vi "Drive Motor TXRX.vi"(0 "Error In":errorcluster, 1 "Speed Control (m/s)":dbl, 3 "RPM / Speed":bool, 5 "Drive Motor Handle In":T2, 7 "Tasking Period":dbl, 9 "RPM Control (rad/s)":dbl, 11 "Controller Data In":refnum<data-value>, 12 "?":T3={"Accelerometer Bias"={"X (m/s)"=0.0, "Y (m/s)"=0.0, "Z (m/s)"=0.0}, "Gyroscope Bias"={"X (m/s)"=0.0, "Y (m/s)"=0.0, "Z (m/s)"=0.0}, "Steering Motor Gear Ratio"=611.0, "Steering Pully Gear Ratio"=1.0, "Steering Encoder CPR"=500.0, "Steering Motor Max RPM"=4000.0, "Wheelbase (m)"=1.12, "Fork Angle (rad)"=1.3, "Balancing Controller"={"Kp (/s)"=0.0, "Kd (1)"=0.0}, "Max Allowed Steering Angle (rad)"=0.7, "Task Periods"={"Emergency Stop (us)"=0, "IMU (us)"=0, "Steering Motor Encoder (us)"=0, "State Estimator (us)"=0, "Balancing Controller (us)"=0, "GNSS (us)"=0, "Logging (us)"=0, "Drive Motor (us)"=0, "Visualization (us)"=50000}, "Drive Motor Gear Ratio"=0.7, "lr"=0.0, "lf"=0.0, "lambda"=0.0, "k1"=0.0, "k2"=0.0, "e1_max"=0.0, "Ad_t"=0.0, "Bd_t"=0.0, "C_t"=0.0, "D_t"=0.0, "Wheel radius"=0.311}, 13 "Ki":dbl, 14 "Kp":dbl) -> (4 "Error Out":errorcluster, 6 "Drive Motor Handle Out":T2, 10 "Drive Motor Data":T1, 15 "Controller Data Out":refnum<data-value>)   [LabVIEW 2021]
uses:
  Drive Motor Handle.ctl
  Configuration/Configuration.ctl
  Drive Motor Data.ctl
  Logging/Controller Data.ctl
  Steering Motor/Steering Motor Data.ctl
panel:
  out "0, 1":i16
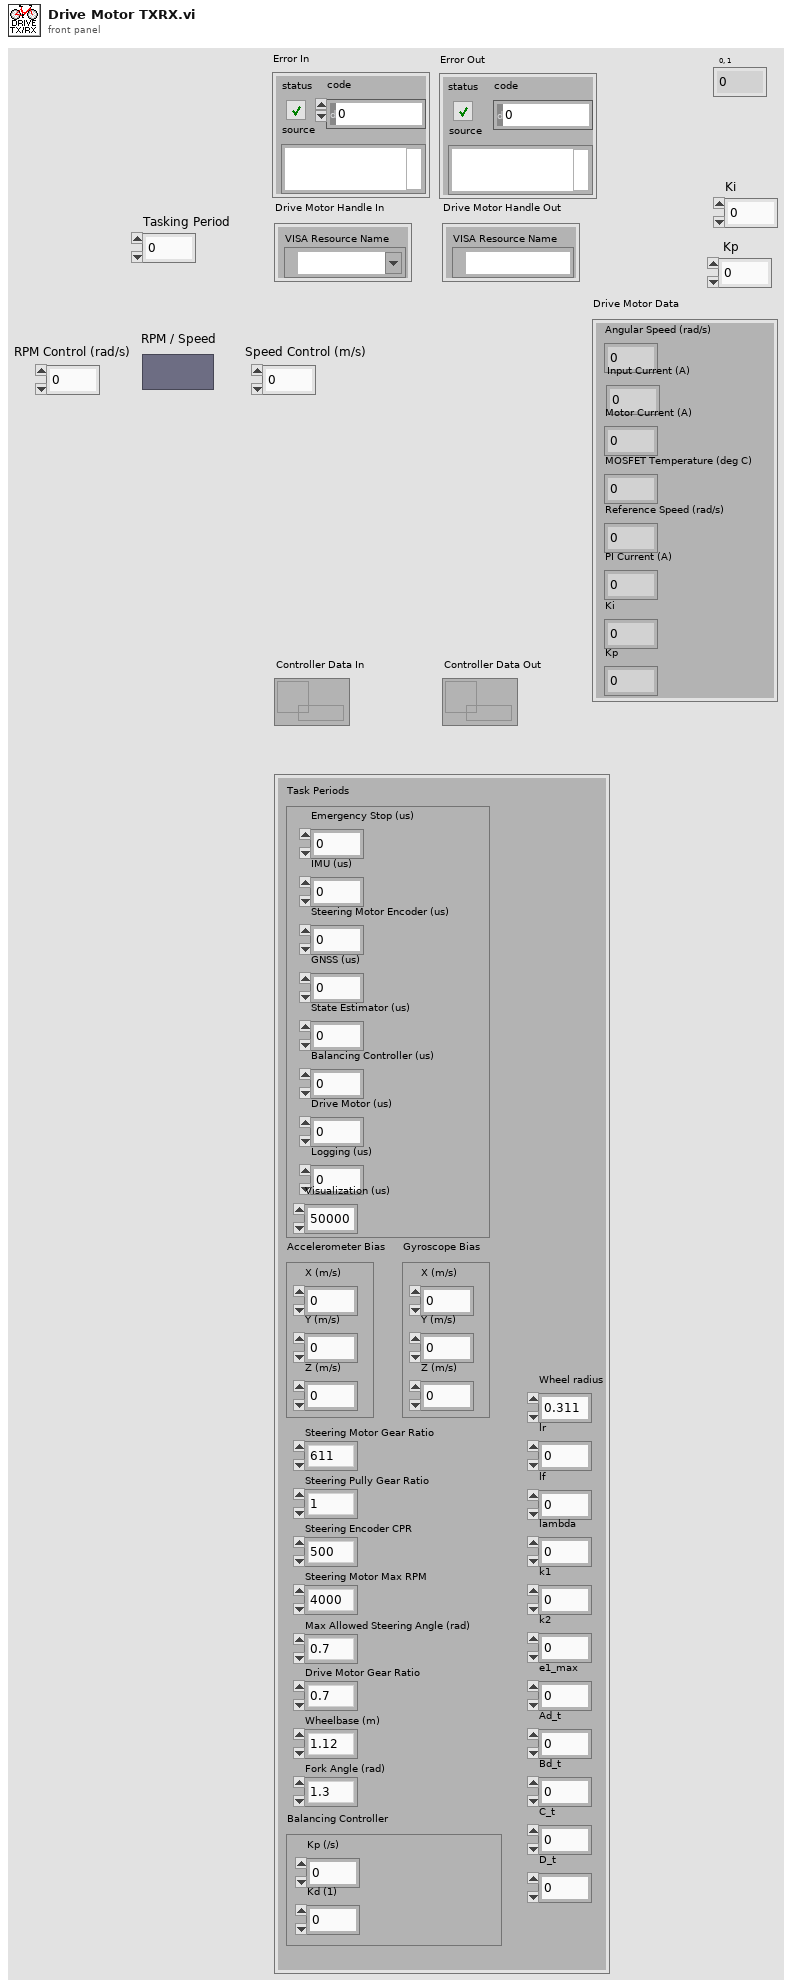
[diagram p1: front panel]
types:
  T1 = typedef "Drive Motor Data.ctl" = cluster{"Angular Speed (rad/s)":dbl, "Input Current (A)":dbl, "Motor Current (A)":dbl, "MOSFET Temperature (deg C)":dbl, "Reference Speed (rad/s)":dbl, "PI Current (A)":dbl, "Ki":dbl, "Kp":dbl}
  T2 = typedef "Drive Motor Handle.ctl" = cluster{"VISA Resource Name":refnum<visa-resource-name>}
  T3 = typedef "Configuration.ctl" = cluster{"Accelerometer Bias":cluster{"X (m/s)":dbl, "Y (m/s)":dbl, "Z (m/s)":dbl}, "Gyroscope Bias":cluster{"X (m/s)":dbl, "Y (m/s)":dbl, "Z (m/s)":dbl}, "Steering Motor Gear Ratio":dbl, "Steering Pully Gear Ratio":dbl, "Steering Encoder CPR":dbl, "Steering Motor Max RPM":dbl, "Wheelbase (m)":dbl, "Fork Angle (rad)":dbl, "Balancing Controller":cluster{"Kp (/s)":dbl, "Kd (1)":dbl}, "Max Allowed Steering Angle (rad)":dbl, "Task Periods":cluster{"Emergency Stop (us)":i64, "IMU (us)":i64, "Steering Motor Encoder (us)":i64, "State Estimator (us)":i64, "Balancing Controller (us)":i64, "GNSS (us)":i64, "Logging (us)":i64, "Drive Motor (us)":i64, "Visualization (us)":i64}, "Drive Motor Gear Ratio":dbl, "lr":dbl, "lf":dbl, "lambda":dbl, "k1":dbl, "k2":dbl, "e1_max":dbl, "Ad_t":dbl, "Bd_t":dbl, "C_t":dbl, "D_t":dbl, "Wheel radius":dbl}
  T4 = typedef "Controller Data.ctl" = cluster{"Drive Motor Data":T1, "Steering Motor Data":T5}
  T5 = typedef "Steering Motor Data.ctl" = cluster{"PWM":dbl, "Steering Angle Rate (rad/s)":dbl, "input balancing":dbl}
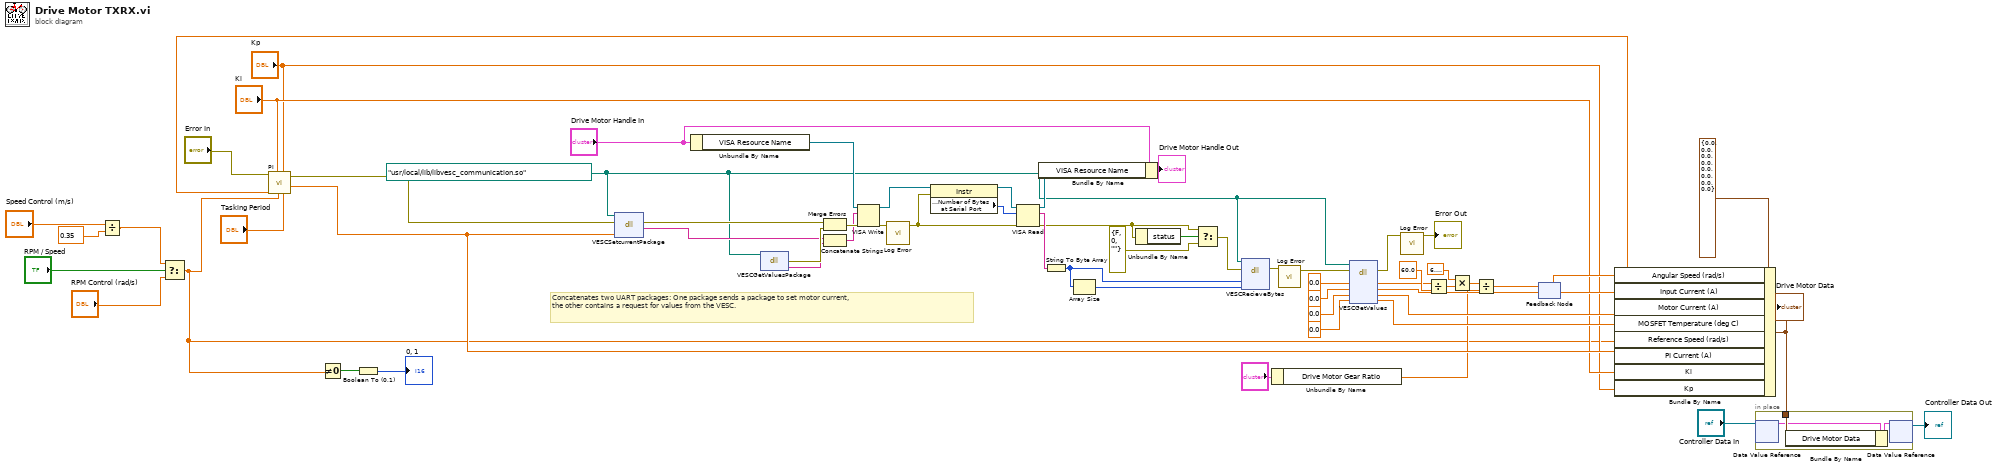
[diagram p0: block diagram]
diagram:
  w16 = path "/usr/local/lib/libvesc_communication.so" ("path in")
  # "Concatenates two UART packages: One package sends a package to set motor current,\nthe other contains a request for values from the VESC."
  n1 = Divide(x="Speed Control (m/s)", y=0.35) -> (x/y=w9:dbl)
  n2 = Select(t=w9, s="RPM / Speed", f="RPM Control (rad/s)") -> (s? t:f=w1:dbl)
  n3 = Not Equal To 0?(x=w1) -> (x != 0?=w20:bool)
  n4 = Boolean To (0,1)(Boolean=w20) -> (0, 1=→"0, 1":i16)
  n5 = Unbundle By Name("Drive Motor Handle In") -> ("VISA Resource Name"=w57:refnum<visa-resource-name>)
  n6 = dll-call lib="?" fn="VESCGetValuesPackage"(path in=w16) -> (error out=w56:errorcluster, "Package"=w22:string)  [unwired: 2 in, 1 out]
  n7 = Unbundle By Name("?") -> ("Drive Motor Gear Ratio"=w4:dbl)
  n8 = feedback #1() -> (w13:dbl)  [unwired: 1 in]
  n9 = call "PI.vi"("Tasking Period"="Tasking Period", "Kp"="Kp", "Reference Speed (rad/s)"=w1, "Ki"="Ki", "Real Speed (rad/s)"=w13, "Error In"="Error In") -> ("PI Current (A)"=w5:dbl, "Error Out"=w12:errorcluster)  [unwired: 4 in]
  n10 = dll-call lib="?" fn="VESCSetcurrentPackage"(path in=w16, error in=w12, "current"=w5) -> (error out=w17:errorcluster, "Package"=w18:string)  [unwired: 2 in, 1 out]
  n11 = Merge Errors(w17, w56) -> (w55:errorcluster)
  n12 = Concatenate Strings(w18, w22) -> (w21:string)
  n13 = VISA Write(VISA resource name=w57, write buffer=w21, error in (no error)=w55) -> (VISA resource name out=w54:refnum<visa-resource-name>, error out=w60:errorcluster)  [unwired: 1 out]
  n14 = call "Log Error.vi"("Error In"=w60) -> ("Error Out"=w42:errorcluster)  [unwired: 10 in]
  n15 = property on="Property Node" class="Instr"(reference=w54, error in=w42) -> (reference out=w49:refnum<visa-resource-name>, "Serial Settings:Number of Bytes at Serial Port"=w52:u32)  [unwired: 1 out]
  n16 = VISA Read(VISA resource name=w49, byte count=w52, error in (no error)=w42) -> (VISA resource name out=w53:refnum<visa-resource-name>, read buffer=w51:string, error out=w50:errorcluster)  [unwired: 1 out]
  n17 = Bundle By Name(cluster="Drive Motor Handle In", "VISA Resource Name"=w53) -> (→"Drive Motor Handle Out":T2)
  n18 = String To Byte Array(string=w51) -> (unsigned byte array=w47:u8[])
  n19 = Array Size(array=w47) -> (size(s)=w48:i32)
  n20 = Unbundle By Name(w50) -> ("status"=w46:bool)
  n21 = Select(t=w50, s=w46, f=errorcluster {"status"=FALSE, "code"=0, "source"=""}) -> (s? t:f=w45:errorcluster)
  n22 = dll-call lib="?" fn="VESCRecieveBytes"(path in=w16, error in=w45, "bytes"=w47, "length"=w48) -> (error out=w43:errorcluster)  [unwired: 4 in, 1 out]
  n23 = call "Log Error.vi"("Error In"=w43) -> ("Error Out"=w23:errorcluster)  [unwired: 10 in]
  n24 = dll-call lib="?" fn="VESCGetValues"(path in=w16, error in=w23, "RPM"=0.0, "currentIn"=0.0, "currentMotor"=0.0 ("RPM"), "tempMOS"=0.0 ("currentIn")) -> (error out=w33:errorcluster, "RPM"=w31:dbl, "currentIn"=w30:dbl, "currentMotor"=w35:dbl, "tempMOS"=w24:dbl)  [unwired: 2 in, 1 out]
  n25 = call "Log Error.vi"("Error In"=w33) -> ("Error Out"=→"Error Out":errorcluster)  [unwired: 10 in]
  n26 = Divide(x=w31, y=60.0 ("x")) -> (x/y=w37:dbl)
  n27 = Multiply(x=6.283185307179586, y=w37) -> (x*y=w29:dbl)
  n28 = Divide(x=w29, y=w4) -> (x/y=w14:dbl)
  n29 = feedback-in #1(w14) -> ()
  n30 = Bundle By Name(cluster=T1 {"Angular Speed (rad/s)"=0.0, "Input Current (A)"=0.0, "Motor Current (A)"=0.0, "MOSFET Temperature (deg C)"=0.0, "Reference Speed (rad/s)"=0.0, "PI Current (A)"=0.0, "Ki"=0.0, "Kp"=0.0} ("Drive Motor Data"), "Angular Speed (rad/s)"=w13, "Input Current (A)"=w30, "Motor Current (A)"=w35, "MOSFET Temperature (deg C)"=w24, "Reference Speed (rad/s)"=w1, "PI Current (A)"=w5, "Ki"="Ki", "Kp"="Kp") -> (w26:T1)
  "Drive Motor Data" <- w26
  n31 = in-place {
    in-place-border: w26 -> [w63]
    n32 = in-place-dvr #2("Controller Data In") -> (w62:T4)  [unwired: 1 out]
    n33 = Bundle By Name(cluster=w62, "Drive Motor Data"=w63) -> (w64:T4)
    n34 = in-place-dvr #2(w64) -> (→"Controller Data Out":refnum<data-value>)  [unwired: 1 out]
  }
